vi "v_grad_rotmatrix.vi"(1 "grad_xyz":dbl[](array[numeric])=[0.0, 0.0, 0.0]) -> (0 "rotate matrix":dbl[][](array[numeric])=[[1.0, 0.0, 0.0, 0.0], [0.0, 1.0, 0.0, 0.0], [0.0, 0.0, 1.0, 0.0], [0.0, 0.0, 0.0, 1.0]] format="%#.2f")   [LabVIEW 2011]
uses:
  <vilib>/Analysis/baseanly.llb/Real A x B.vi
  <vilib>/Analysis/NI_AALBase.lvlib
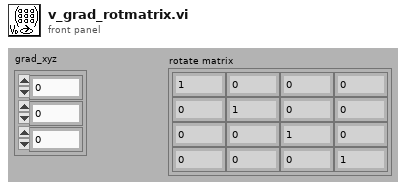
[diagram p1: front panel]
types:
  T1 = cluster{"grad_xyz[0]":dbl, "grad_xyz[1]":dbl, "grad_xyz[2]":dbl}
  T2 = typedef "NI_Matrix.lvlib/RealMatrix.ctl" = dbl[][]
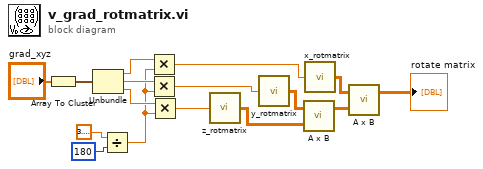
[diagram p0: block diagram]
diagram:
  n1 = Array To Cluster(array="grad_xyz") -> (cluster=w11:T1)
  n2 = Unbundle(w11) -> ("grad_xyz[0]"=w3:dbl, "grad_xyz[1]"=w5:dbl, "grad_xyz[2]"=w6:dbl)
  n3 = Divide(x=3.141592653589793, y=180) -> (x/y=w1:dbl)
  n4 = Multiply(x=w3, y=w1) -> (x*y=w2:dbl)
  n5 = Multiply(x=w5, y=w1) -> (x*y=w4:dbl)
  n6 = Multiply(x=w6, y=w1) -> (x*y=w7:dbl)
  n7 = call "z_rotmatrix.vi"("z-angle"=w7) -> ("z-matrix"=w13:dbl[][])
  n8 = call "y_rotmatrix.vi"("y-angle"=w4) -> ("y-matrix"=w16:dbl[][])
  n9 = call-poly <vilib>:"A x B.vi"("B"=w13, "A"=w16) -> ("A x B"=w15:T2)  [unwired: 1 out]
  n10 = call "x_rotmatrix.vi"("x-angle"=w2) -> ("x-matrix"=w14:dbl[][])
  n11 = call-poly <vilib>:"A x B.vi"("B"=w15, "A"=w14) -> ("A x B"=→"rotate matrix":T2)  [unwired: 1 out]
